vi "CallDisplayData.vi"(2 "Data":variant) -> ()   [LabVIEW 2020]
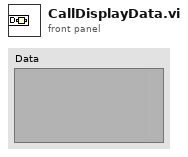
[diagram p1: front panel]
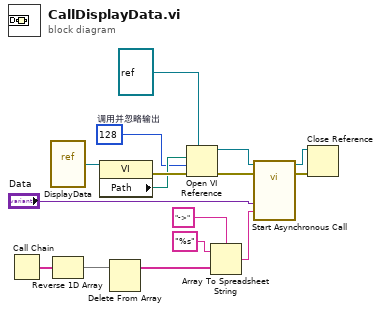
[diagram p0: block diagram]
diagram:
  w3 = 128  # 调用并忽略输出
  n1 = Call Chain() -> (call chain=w11:string[])
  n2 = vi-ref "DisplayData.vi"() -> (w8:refnum<vi>)
  n3 = Reverse 1D Array(array=w11) -> (reversed array=w2:string[])
  n4 = property class="VI"(reference=w8) -> (error out=w10:errorcluster, "Path"=w9:path)  [unwired: 1 in, 1 out]
  n5 = Delete From Array(array=w2) -> (array with subset deleted=w1:string[])  [unwired: 2 in, 1 out]
  n6 = Open VI Reference(type specifier VI Refnum (for type only)=refnum<vi> refnum, vi path=w9, options=w3, error in (no error)=w10) -> (vi reference=w4:refnum<vi>, error out=w5:errorcluster)  [unwired: 2 in]
  n7 = Array To Spreadsheet String(delimiter (Tab)="->" ("分隔符(Tab)"), array=w1, 3:"%s" ("格式字符串")) -> (spreadsheet string=w14:string)
  n8 = call-by-ref "Start Asynchronous Call"(reference=w4, error in=w5, "前面板窗口:标题"=w14, "变体"="Data") -> (reference out=w7:refnum<vi>, error out=w6:errorcluster)  [unwired: 10 in]
  n9 = Close Reference(reference=w7, error in (no error)=w6) -> ()  [unwired: 1 out]
